vi "AMC QR Get Queue .vi"(8 "error in (no error)":errorcluster, 11 "Name":string) -> (0 "error out":errorcluster, 3 "Queue Out":T1)   [LabVIEW 2017]
doc: "This VI removes the host connection from the connection manager list if it becomes disconnected for any reason."
uses:
  TypeDefs/amc_QueueRegistryMethod.ctl
  TypeDefs/amc_QueueRegistryProperties.ctl
  subVIs/TypeDefs/amc_Message.ctl
  subVIs/TypeDefs/amc_Message Queue.ctl
  Tools/Keyed Array/Tools_KeyedArray KeyedArray.ctl
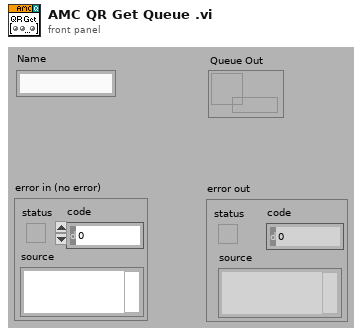
[diagram p1: front panel]
types:
  T1 = typedef "amc_Message Queue.ctl" = refnum<queue>
  T2 = typedef "amc_QueueRegistryProperties.ctl" = cluster{"Name":string}
  T3 = typedef "amc_QueueRegistryMethod.ctl" = enum16{"Initialize", "Add Queue", "Set Properties", "Get Queue by Index", "Get Queue by Name", "Remove Queue", "Remove All Queues"}
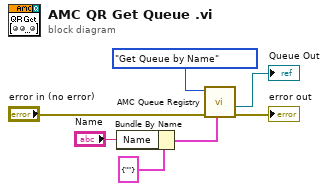
[diagram p0: block diagram]
diagram:
  n1 = Bundle By Name(cluster=T2 {"Name"=""} ("Properties In"), "Name"="Name") -> (w4:T2)
  n2 = call "AMC Queue Registry.vi"("Properties in"=w4, "error in (no error)"="error in (no error)", "Method"=amc_QueueRegistryMethod."Get Queue by Name") -> ("error out"=→"error out":errorcluster, "Message Queue out"=→"Queue Out":T1)  [unwired: 2 in, 5 out]
